vi "GetModuleIndex.vi"(11 "ModuleType":string) -> (3 "ModuleIndex":i32, 5 "Error":errorcluster)   [LabVIEW 2014, in "Test.lvclass"]
uses:
  Test.lvclass
  <vilib>/Utility/error.llb/Error Cluster From Error Code.vi
  <vilib>/ErrorRing/Error Ring.xnode
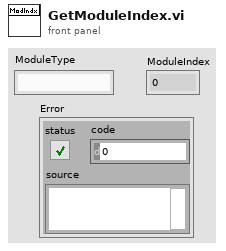
[diagram p1: front panel]
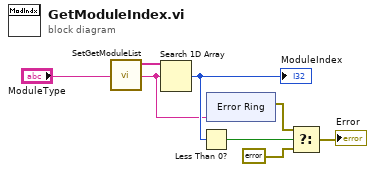
[diagram p0: block diagram]
diagram:
  n1 = call "SetGetModuleList.vi"() -> ("ModuleList"=w7:string[])  [unwired: 11 in]
  n2 = Search 1D Array(1D array=w7, element="ModuleType") -> (index of element=w6:i32)  [unwired: 1 in]
  "ModuleIndex" <- w6
  n3 = Less Than 0?(x=w6) -> (x < 0?=w5:bool)
  n4 = xnode "Error Ring"("parameter 0"="ModuleType") -> ("error out"=w4:errorcluster)
  n5 = Select(t=w4, s=w5, f=errorcluster {"status"=FALSE, "code"=0, "source"=""}) -> (s? t:f=→"Error":errorcluster)
